vi "Get SLSC Modules Section.vi"(8 "error in (no error)":errorcluster, 11 "SLSC Chassis":refnum<k24>) -> (0 "error out":errorcluster, 2 "Modules Section":refnum<k24>, 3 "SLSC Chassis out":refnum<k24>)   [LabVIEW 2017, in "VeriStand SLSC Scripting.lvlib"]
uses:
  VeriStand SLSC Scripting.lvlib
  NationalInstruments.VeriStand.SystemDefinitionAPI
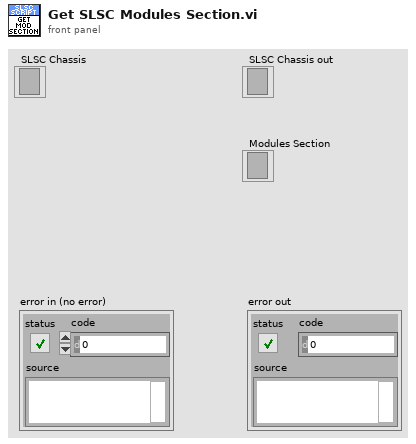
[diagram p1: front panel]
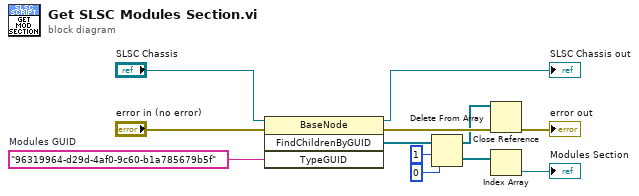
[diagram p0: block diagram]
diagram:
  w12 = "96319964-d29d-4af0-9c60-b1a785679b5f"  # Modules GUID
  n1 = invoke class="BaseNode" method="FindChildrenByGUID"(reference="SLSC Chassis", error in="error in (no error)", "TypeGUID"=w12) -> (reference out=→"SLSC Chassis out":refnum<k24>, error out=w6:errorcluster, "FindChildrenByGUID"=w9:refnum<k24>[])  [unwired: 1 in, 1 out]
  n2 = Delete From Array(array=w9, length=1, index=0) -> (deleted portion=w4:refnum<k24>[], array with subset deleted=w5:refnum<k24>[])
  n3 = Close Reference(reference=w5, error in (no error)=w6) -> (error out=→"error out":errorcluster)
  n4 = Index Array(array=w4) -> (element=→"Modules Section":refnum<k24>)  [unwired: 1 in]
